vi "DFD Narrowband Filtering (Array).vi"(7 "init? (F)":bool, 8 "error in (no error)":errorcluster, 10 "narrowband filter":T1 {"multirate filters"."mMRate_SumWl" min=1 max=32 step=1; "multirate filters"."mMRate_InputIwl" min=1 max=32 step=1; "multirate filters"."mMRate_GainWl" min=1 max=32 step=1; "multirate filters"."mMRate_OutputWl" min=1 max=32 step=1; "multirate filters"."mMRate_InputWl" min=1 max=32 step=1; "multirate filters"."mMRate_CoefWl" min=1 max=32 step=1; "multirate filters"."mMRate_Mode" items=["Default"=-1, "No Rate Change"=0, "Interpolation"=1, "Decimation"=2, "Interpolated"=3, "Rational"=4]}, 11 "signal in":dbl[](array[numeric])) -> (0 "error out":errorcluster, 3 "signal out":dbl[](array[numeric]))   [LabVIEW 2017, in "NI_DigFilterLicensed.lvlib"]
doc: "Filters a signal continuously with a narrowband filter. Wire data to the <B>signal in</B> input to determine the polymorphic instance to use or manually select the instance."
uses:
  <vilib>/addons/Digital Filter Design/NI_DigFilterLicensed.lvlib
  <vilib>/addons/Digital Filter Design/_Objects.llb/DFD Narrowband Filter Obj.ctl
  <vilib>/addons/Digital Filter Design/_Objects.llb/DFD Multirate Filter Obj.ctl
  <vilib>/addons/Digital Filter Design/_Objects.llb/DFD Multirate Mode.ctl
  <vilib>/addons/Digital Filter Design/_Objects.llb/DFD Coef Norm Type.ctl
  <vilib>/addons/Digital Filter Design/_Objects.llb/DFD Round-off Mode.ctl
  <vilib>/addons/Digital Filter Design/_Objects.llb/DFD FXP MRate Multiply Mode.ctl
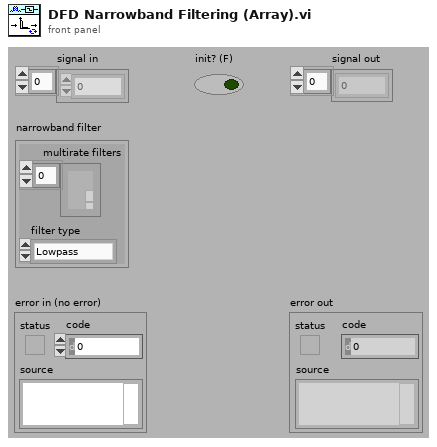
[diagram p1: front panel]
types:
  T1 = typedef "NI_DigFilterLicensed.lvlib/DFD Narrowband Filter Obj.ctl" = cluster{"multirate filters":T2[], "filter type":enum32{"Lowpass", "Highpass", "Bandpass", "Bandstop", "Wideband-Lowpass", "Wideband-Highpass"}}
  T2 = typedef "NI_DigFilterLicensed.lvlib/DFD Multirate Filter Obj.ctl" = cluster{"mMRate_Structure":enum16{"CIC", "FIR", "IIR", "Lattice"}, "mMRate_Mode":T3, "mMRate_Factor":i32, "mMRate_FIRParams":cluster{"mMRate_FIR_H":dbl[], "mMRate_FIR_IsNyquist?":bool, "mMRate_FIR_IsSymmetric?":bool}, "mMRate_CICParams":cluster{"mMRate_CIC_#Stage":i32, "mMRate_CIC_Lag":i32, "mMRate_CIC_Type":enum16{"Lowpass", "Highpass"}}, "mMRate_Order":i32, "mMRate_Version":string, "mMRate_Comments":string, "mMRate_RationalFactor":cluster{"mMRate_L":i32, "mMRate_M":i32}, "mMRate_Fs":dbl, "mMRate_Quantized?":bool, "mMRate_QFilterGain":dbl, "mMRate_CoefWl":i16, "mMRate_Scaling":cluster{"mMRate_ScaleByPowerOf2?":bool, "mMRate_ScaleType":T4}, "mMRate_InputWl":i16, "mMRate_OutputWl":i16, "mMRate_OutputMode":T5, "mMRate_MultMode":T6, "mMRate_BitPruning":bool, "mMRate_GainWl":i16, "mMRate_OutputFwl":i16, "mMRate_SumIwl":i16, "mMRate_InputIwl ":i16, "mMRate_SumWl":i16, "mMRate_CoefIwl":i16}
  T3 = typedef "NI_DigFilterLicensed.lvlib/DFD Multirate Mode.ctl" = i16
  T4 = typedef "NI_DigFilterLicensed.lvlib/DFD Coef Norm Type.ctl" = enum16{"No Norm", "Time Domain 1-Norm", "Time Domain 2-Norm", "Time Domain Inf-Norm"}
  T5 = typedef "NI_DigFilterLicensed.lvlib/DFD Round-off Mode.ctl" = enum16{"Nearest", "Truncation"}
  T6 = typedef "NI_DigFilterLicensed.lvlib/DFD FXP MRate Multiply Mode.ctl" = enum16{"Truncated", "Full"}
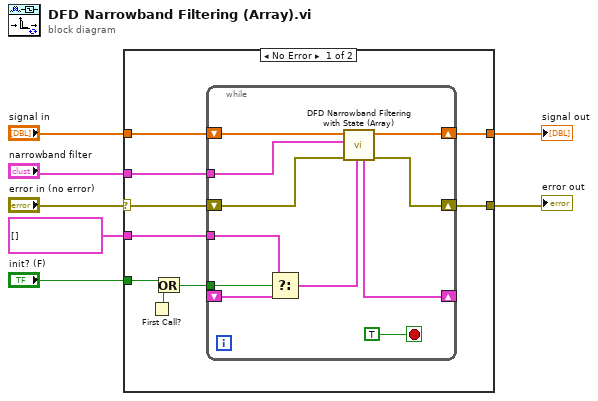
[diagram p0: block diagram]
diagram:
  n1 = case shown="No Error" "error in (no error)" {
    selector: "error in (no error)" -> [w14 w29]
    tunnel: [w13 w29] -> w6
    tunnel: "signal in" -> [w16 w28]
    tunnel: [w15 w28] -> w4
    tunnel: cluster{"state out":dbl[]}[] [] ("state in") -> [w12 _]
    tunnel: "narrowband filter" -> [w11 _]
    tunnel: "init? (F)" -> [w9 _]
    frame No Error {
      n2 = First Call?() -> (First Call?: T/F=w10:bool)
      n3 = Or(x=w9, y=w10) -> (x .or. y?=w8:bool)
      n4 = while {
        shift-right: [w24] -> _
        shift-left: _ -> [w22]
        tunnel: w8 -> [w20]
        tunnel: w12 -> [w17]
        tunnel: w11 -> [w18]
        shift-right: [w26] -> w15
        shift-left: w16 -> [w27]
        shift-right: [w19] -> w13
        shift-left: w14 -> [w23]
        stop <- TRUE stop-if-true
        n5 = Select(t=w17, s=w20, f=w22) -> (s? t:f=w21:cluster{"state ":dbl[]}[])
        n6 = call <vilib>:"DFD Narrowband Filtering with State (Array).vi"("state in"=w21, "error in (no error)"=w23, "narrowband filter"=w18, "signal in"=w27) -> ("error out"=w19:errorcluster, "signal out"=w26:dbl[], "state out"=w24:cluster{"state ":dbl[]}[])  [unwired: 5 out]
      }
    }
    frame Error {
    }
  }
  "error out" <- w6
  "signal out" <- w4
